vi "PicoScope3000aUnitInfo.vi"(3 "Mode":u16(ring) items=["Dialog On Error", "no dialog - CloseUnit and Stop", "no dialog - Continue", "no dialog - Stop"], 4 "handle in":i16, 5 "error in (no error)":errorcluster) -> (0 "Unit Info":T1, 1 "handle out":i16, 2 "error out":errorcluster)   [LabVIEW 2010]
uses:
  ps3000a.dll
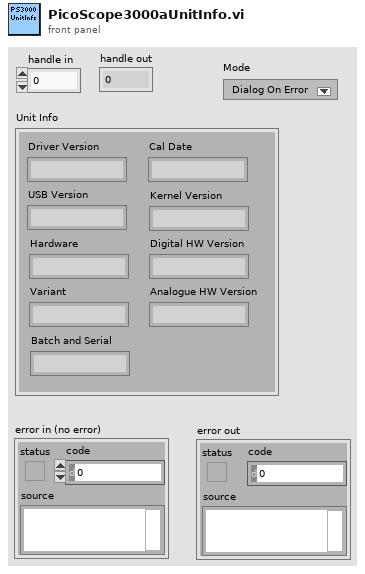
[diagram p1: front panel]
types:
  T1 = cluster{"Driver Version":string, "USB Version":string, "Hardware":string, "Variant":string, "Batch and Serial":string, "Cal Date":string, "Kernel Version":string, "Digital HW Version":string, "Analogue HW Version":string}
  T2 = cluster{"status":bool, "code":u32, "source":string}
  T3 = cluster{"[0]":string, "[1]":string, "[2]":string, "[3]":string, "[4]":string, "[5]":string, "[6]":string, "[7]":string, "[8]":string}
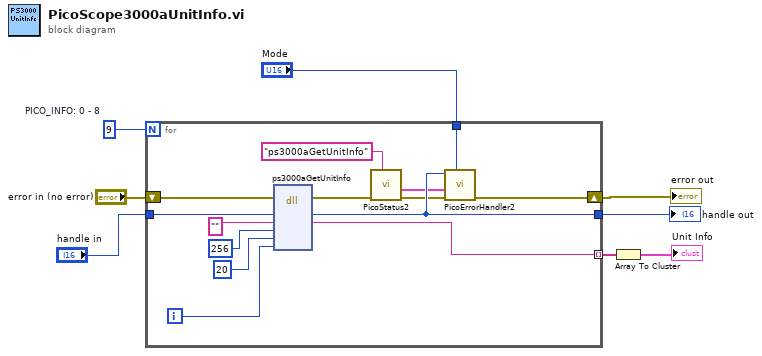
[diagram p0: block diagram]
diagram:
  w7 = 9  # PICO_INFO: 0 - 8
  n1 = for {
    N: w7 -> [_]
    tunnel: "handle in" -> [w22]
    tunnel: [w19] -> w4 mode=indexing
    tunnel: [w14] -> w5
    tunnel: "Mode" -> [w15]
    shift-right: [w13] -> w1
    shift-left: "error in (no error)" -> [w16]
    i -> [w17]
    n2 = dll-call lib="ps3000a.dll" fn="ps3000aGetUnitInfo"(error in=w16, "handle"=w22, "unitInfo"="", "stringLength"=i16 256, "requiredSize"=i16 20 ("stringLength"), "pico_info"=w17) -> (error out=w12:errorcluster, "handle"=w14:i16, "unitInfo"=w19:string)  [unwired: 6 in, 1 out]
    n3 = call "PicoStatus2.vi"("PICO source"="ps3000aGetUnitInfo" ("source"), "Error in"=w12) -> ("error out"=w11:errorcluster, "PICO_STATUS out"=w9:T2)  [unwired: 6 in]
    n4 = call "PicoErrorHandler2.vi"("Mode"=w15, "error in (no error)"=w11, "PICO_STATUS in"=w9, "handle In"=w14) -> ("error out"=w13:errorcluster)  [unwired: 7 in]
  }
  "error out" <- w1
  "handle out" <- w5
  n5 = Array To Cluster(array=w4) -> (cluster=→"Unit Info":T3)
